vi "update digital software pulse .vi"(10 "frequency":i32, 11 "handle":u32) -> (2 "function return":bool, 3 "handle out":u32)   [LabVIEW 2020, in "cDaq.lvlib"]
doc: "DAQAPI bool update_digital_software_pulse_(HDAQ handle, int frequency);"
uses:
  cDaq.lvlib
  cDaq.dll
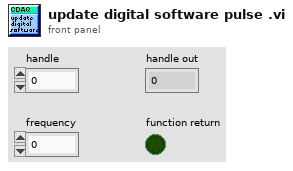
[diagram p1: front panel]
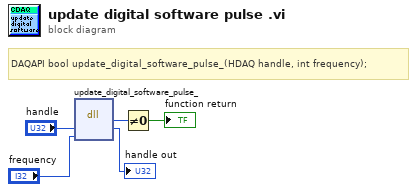
[diagram p0: block diagram]
diagram:
  # "DAQAPI bool update_digital_software_pulse_(HDAQ handle, int frequency);"
  n1 = dll-call lib="G:/CODE/01-Cplusplus/cDaq/doc/UsingWithLabview/cDaqlib/cDaq.*" fn="update_digital_software_pulse_"("handle"="handle", "frequency"="frequency") -> (w4:u8, "handle"=→"handle out":u32)  [unwired: 4 in, 2 out]
  n2 = Not Equal To 0?(x=w4) -> (x != 0?=→"function return":bool)
